vi "Graphs and charts.vi"() -> ()   [LabVIEW 2021]
panel:
  out "Waveform Graph":dbl[](graph)
  in  "?":bool
  out "Temp Value (C)":dbl
  out "Waveform Chart":dbl(graph)
  in  "Thermometer (F)":dbl(slide) scale=0.0..100.0
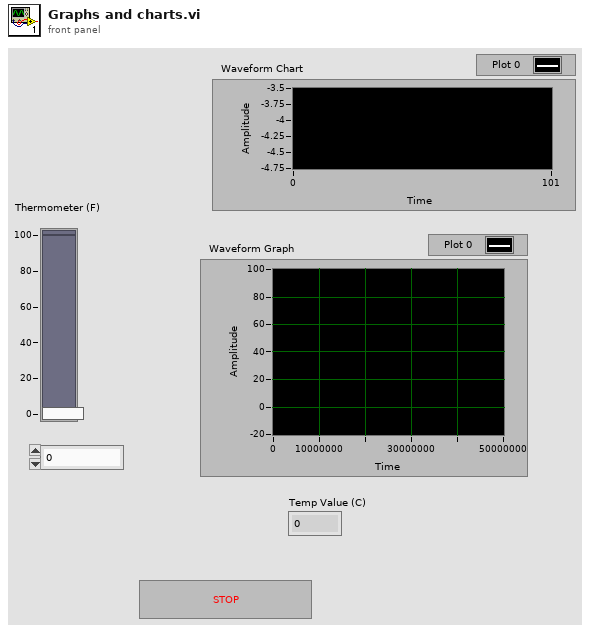
[diagram p1: front panel]
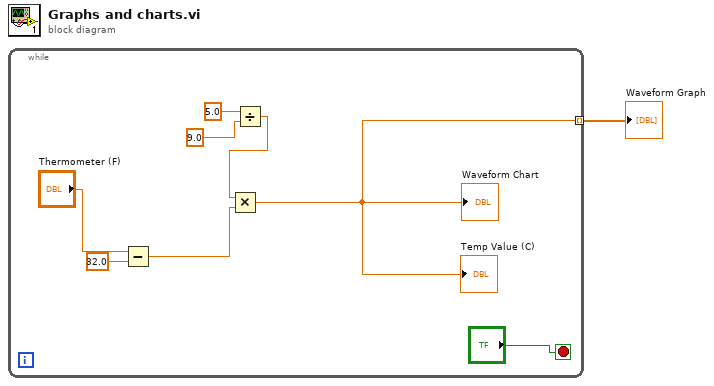
[diagram p0: block diagram]
diagram:
  n1 = while {
    tunnel: [w2] -> w1 mode=indexing
    stop <- "?" stop-if-true
    n2 = Subtract(x="Thermometer (F)", y=32.0) -> (x-y=w8:dbl)
    n3 = Divide(x=5.0, y=9.0) -> (x/y=w7:dbl)
    n4 = Multiply(x=w7, y=w8) -> (x*y=w2:dbl)
    "Waveform Chart" <- w2
    "Temp Value (C)" <- w2
  }
  "Waveform Graph" <- w1
